vi "Day 22-Part 2-Split Cubes.vi"() -> ()   [LabVIEW 2021]
uses:
  <vilib>/regexp/Match Regular Expression.xnode
  <vilib>/Utility/file.llb/Read Delimited Spreadsheet (string).vi
panel:
  out "size(s)":i32[](array[numeric])
  out "Cubes On":i64
  out "Array":cluster{bool, i32[]}[](array[cluster])
  in  "Input File":enum32{"example input", "input"}(radio)
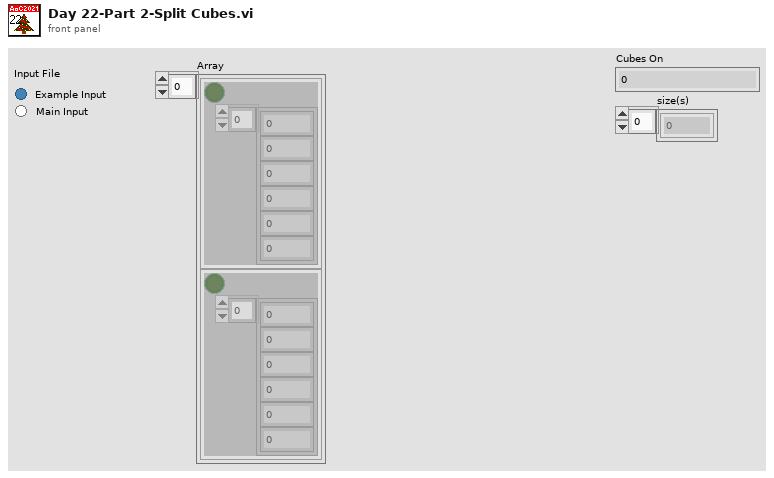
[diagram p1: front panel]
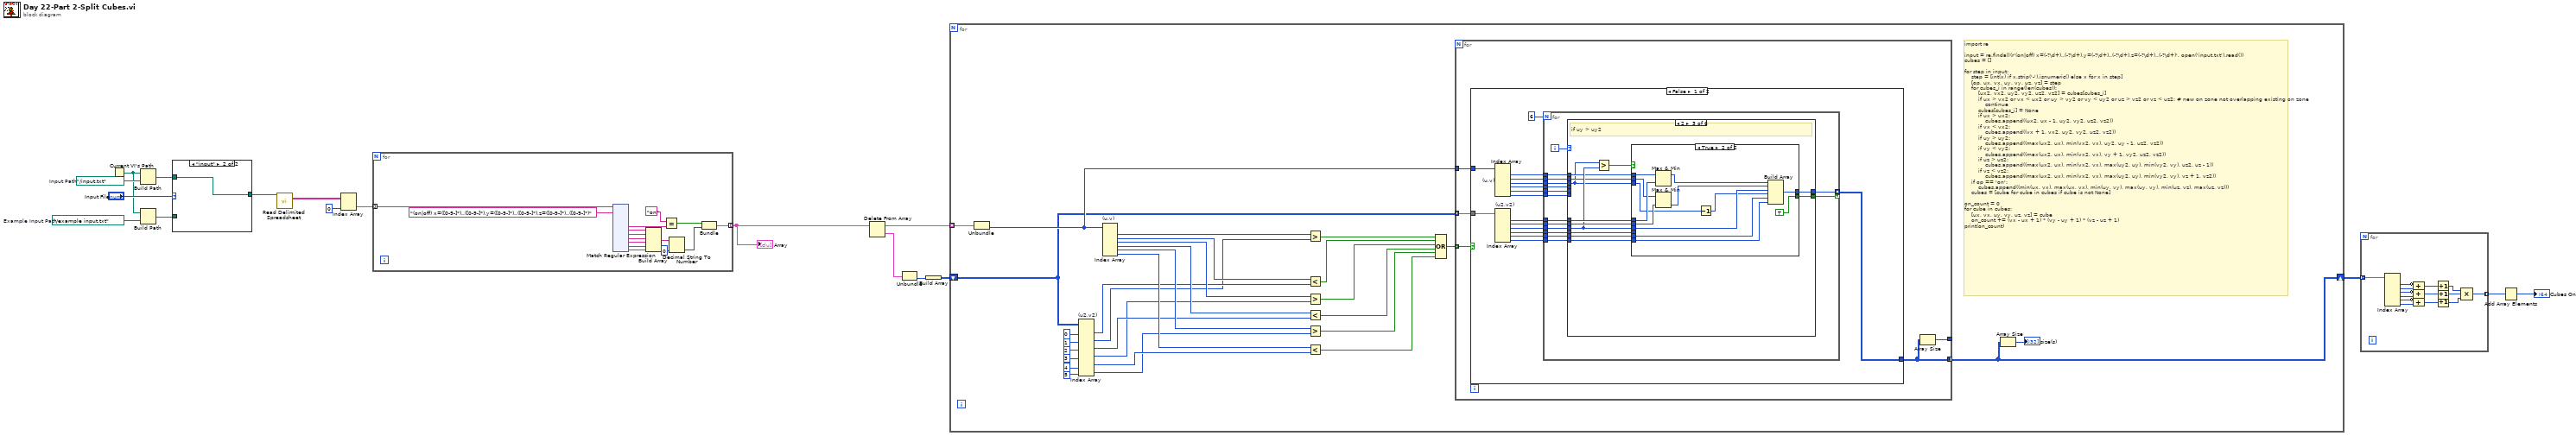
[diagram p0: block diagram]
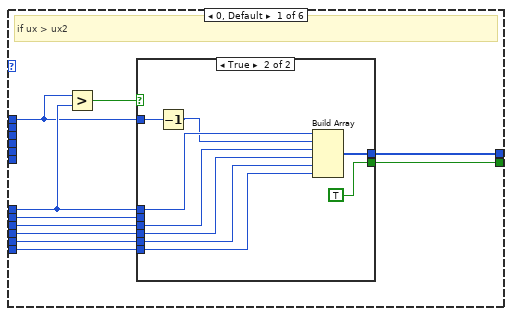
[diagram p2: hidden frame]
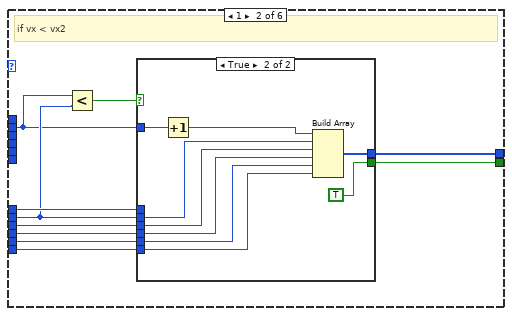
[diagram p4: hidden frame]
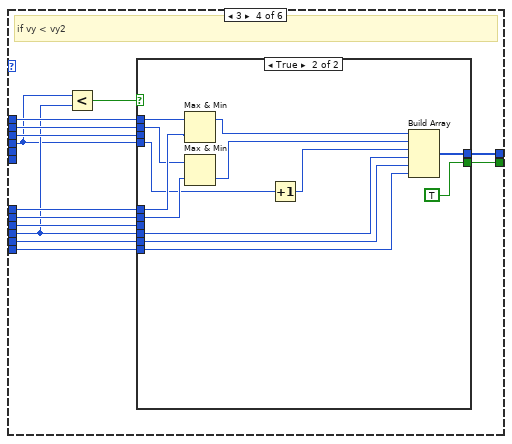
[diagram p7: hidden frame]
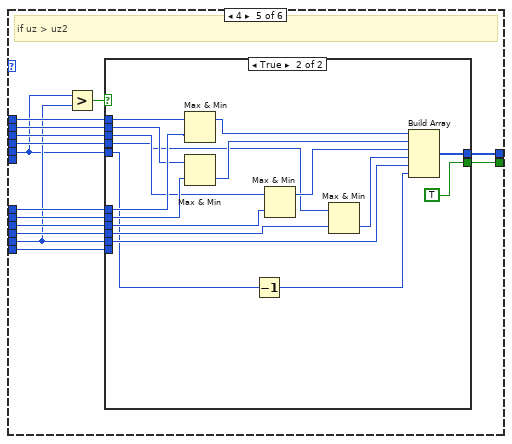
[diagram p9: hidden frame]
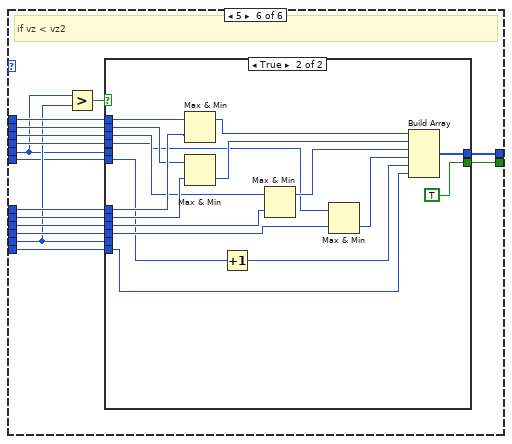
[diagram p11: hidden frame]
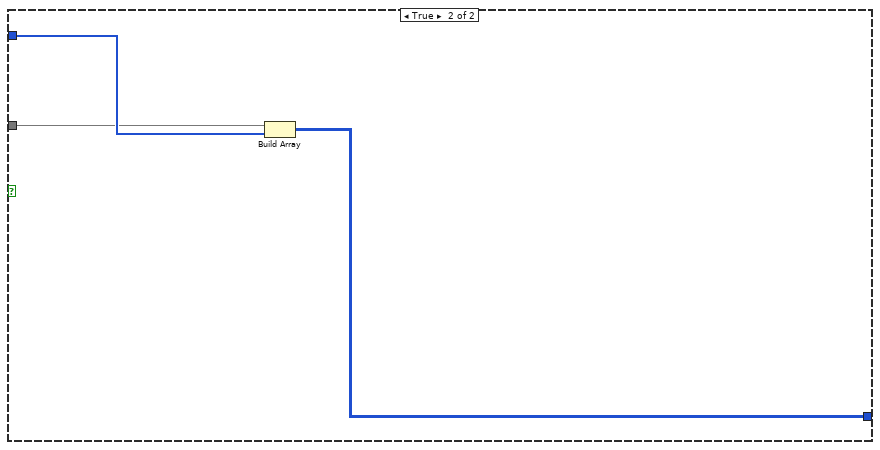
[diagram p13: hidden frame]
diagram:
  w17 = path "../example input.txt"  # Example Input Path
  w18 = path "../input.txt"  # Input Path
  n1 = Current VI's Path() -> (path=w12:path)
  n2 = Build Path(base path=w12, name or relative path=w18) -> (appended path=w15:path)
  n3 = Build Path(base path=w12, name or relative path=w17) -> (appended path=w14:path)
  n4 = case shown="\"input\"" "Input File" {
    tunnel: w15 -> [_ w20]
    tunnel: w14 -> [w19 _]
    tunnel: [w19 w20] -> w13
    frame "example input" {
    }
    frame "input" {
    }
  }
  n5 = call-poly <vilib>:"Read Delimited Spreadsheet.vi"("file path (dialog if empty)"=w13) -> ("all rows"=w11:string[][])  [unwired: 9 in, 5 out]
  n6 = Index Array(array=w11, index (col)=0 ("disabled index (col)")) -> (element=w9:string[])  [unwired: 1 in]
  n7 = for {
    tunnel: w9 -> [w35] mode=indexing
    tunnel: [w23] -> w8 mode=indexing
    n8 = xnode "Match Regular Expression"("input string"=w35, "regular expression"="(on|off) x=([0-9-]*)..([0-9-]*),y=([0-9-]*)..([0-9-]*),z=([0-9-]*)..([0-9-]*)") -> ("submatch 1"=w33:string, "submatch 2"=w30:string, "submatch 3"=w29:string, "submatch 4"=w28:string, "submatch 5"=w27:string, "submatch 6"=w26:string, "submatch 7"=w25:string)  [unwired: 4 in, 5 out]
    n9 = Build Array(w30, w29, w28, w27, w26, w25) -> (w24:string[])
    n10 = Equal?(x="on", y=w33) -> (x = y?=w31:bool)
    n11 = Decimal String To Number(string=w24, default (0L)=i64 0 ("default (0 I32)")) -> (number=w22:i64[])  [unwired: 1 in, 1 out]
    n12 = Bundle(w31, w22) -> (w23:cluster{bool, i64[]})  [unwired: 1 in]
  }
  "Array" <- w8
  n13 = Delete From Array(array=w8) -> (deleted portion=w6:cluster{bool, i64[]}, array with subset deleted=w7:cluster{bool, i64[]}[])  [unwired: 2 in]
  n14 = Unbundle(w6) -> (w5:i64[])  [unwired: 1 out]
  n15 = Build Array(w5) -> (w4:i64[][])
  n16 = for {
    tunnel: w7 -> [w190] mode=indexing
    shift-right: [w162] -> w3
    shift-left: w4 -> [w188]
    # "import re\n\ninput = re.findall(r'(on|off) x=(-?\\d+)..(-?\\d+),y=(-?\\d+)..(-?\\d+),z=(-?\\d+)..(-?\\d+)', open('input.txt').read())\ncubes = []\n\nfor step in input:\n    step = [int(x) if x.strip('-').isnumeric() else x for x in step]\n    [op, ux, vx, uy, vy, uz, vz] = step\n    for cubes_i in range(len(cubes)):\n        [ux2, vx2, uy2, vy2, uz2, vz2] = cubes[cubes_i]\n        if ux > vx2 or vx < ux2 or uy > vy2 or vy < uy2 or uz > vz2 or vz < uz2: # new on zone not overlapping existing on zone\n            continue\n        cubes[cubes_i] = None\n        if ux > ux2:\n            cubes.append((ux2, ux - 1, uy2, vy2, uz2, vz2))\n        if vx < vx2:\n            cubes.append((vx + 1, vx2, uy2, vy2, uz2, vz2))\n        if uy > uy2:\n            cubes.append((max(ux2, ux), min(vx2, vx), uy2, uy - 1, uz2, vz2))\n        if vy < vy2:\n            cubes.append((max(ux2, ux), min(vx2, vx), vy + 1, vy2, uz2, vz2))\n        if uz > uz2:\n            cubes.append((max(ux2, ux), min(vx2, vx), max(uy2, uy), min(vy2, vy), uz2, uz - 1))\n        if vz < vz2:\n            cubes.append((max(ux2, ux), min(vx2, vx), max(uy2, uy), min(vy2, vy), vz + 1, vz2))\n    if op == 'on':\n        cubes.append((min(ux, vx), max(ux, vx), min(uy, vy), max(uy, vy), min(uz, vz), max(uz, vz)))\n    cubes = [cube for cube in cubes if cube is not None]\n\non_count = 0\nfor cube in cubes:\n    [ux, vx, uy, vy, uz, vz] = cube\n    on_count += (vx - ux + 1) * (vy - uy + 1) * (vz - uz + 1)\nprint(on_count)"
    n17 = Unbundle(w190) -> (w189:i64[])  [unwired: 1 out]
    n18 = Index Array "(u2,v2)"(array=w188, index (col) #1=0 ("disabled index (col)"), index (col) #2=1 ("index (col)"), index (col) #3=2 ("index (col)"), index (col) #4=3 ("index (col)"), index (col) #5=4 ("index (col)"), index (col) #6=5 ("index (col)")) -> (element #1=w169:i64[], element #2=w168:i64[], element #3=w167:i64[], element #4=w166:i64[], element #5=w165:i64[], element #6=w164:i64[])  [unwired: 6 in]
    n19 = Index Array "(u,v)"(array=w189) -> (element #1=w187:i64, element #2=w185:i64, element #3=w183:i64, element #4=w181:i64, element #5=w179:i64, element #6=w178:i64)  [unwired: 6 in]
    n20 = Greater?(x=w187, y=w168) -> (0:w186:bool[])
    n21 = Less?(x=w185, y=w169) -> (x < y?=w184:bool[])
    n22 = Greater?(x=w183, y=w166) -> (0:w182:bool[])
    n23 = Less?(x=w181, y=w167) -> (x < y?=w180:bool[])
    n24 = Greater?(x=w179, y=w164) -> (0:w177:bool[])
    n25 = Less?(x=w178, y=w165) -> (x < y?=w176:bool[])
    n26 = Compound Arithmetic op=OR(w186, w184, w182, w180, w177, w176) -> (w163:bool[])
    n27 = for {
      tunnel: w189 -> [w195]
      tunnel: w188 -> [w194] mode=indexing
      tunnel: [w192] -> w162 mode=concatenating
      tunnel: w163 -> [w193] mode=indexing
      tunnel: [w191] -> _
      n28 = case shown="False" w193 {
        tunnel: w195 -> [w211 w381]
        tunnel: [w196 w380] -> w192
        tunnel: w194 -> [w210 w379]
        frame False {
          n29 = Index Array "(u,v)"(array=w211) -> (element #1=w209:i64, element #2=w201:i64, element #3=w200:i64, element #4=w199:i64, element #5=w198:i64, element #6=w197:i64)  [unwired: 6 in]
          n30 = Index Array "(u2,v2)"(array=w210) -> (element #1=w207:i64, element #2=w208:i64, element #3=w206:i64, element #4=w205:i64, element #5=w204:i64, element #6=w203:i64)  [unwired: 6 in]
          n31 = for {
            N: 6 -> [_]
            tunnel: w209 -> [w226]
            tunnel: w208 -> [w225]
            tunnel: w207 -> [w224]
            tunnel: w206 -> [w223]
            tunnel: w205 -> [w222]
            tunnel: w204 -> [w221]
            tunnel: w203 -> [w220]
            tunnel: w201 -> [w216]
            tunnel: w200 -> [w215]
            tunnel: w199 -> [w214]
            tunnel: w198 -> [w213]
            tunnel: w197 -> [w212]
            tunnel: [w218] -> w196 mode=indexing if=w217
            i -> [w219]
            n32 = case shown="2" w219 {
              tunnel: w226 -> [w229 _ w267 w294 w322 w354]
              tunnel: w225 -> [w235 w247 w269 w296 w324 w356]
              tunnel: w224 -> [w234 w254 w275 w301 w328 w360]
              tunnel: w223 -> [w233 w253 w268 w295 w323 w355]
              tunnel: w222 -> [w232 w252 w274 w291 w319 w351]
              tunnel: w221 -> [w231 w251 w273 w300 w317 w349]
              tunnel: w220 -> [w230 w250 w272 w299 w327 w359]
              tunnel: [w228 w249 w271 w298 w326 w358] -> w218
              tunnel: [w227 w248 w270 w297 w325 w357] -> w217
              tunnel: w216 -> [_ w246 w266 w293 w321 w353]
              tunnel: w215 -> [_ _ w265 w292 w320 w352]
              tunnel: w214 -> [_ _ _ w290 w318 w350]
              tunnel: w213 -> [_ _ _ _ w316 w348]
              tunnel: w212 -> [_ _ _ _ _ w347]
              frame 0, Default {
                # "if ux > ux2"
                n33 = Greater?(x=w229, y=w234) -> (0:w236:bool)
                n34 = case shown="True" w236 {
                  tunnel: w235 -> [_ _]
                  tunnel: w234 -> [_ w245]
                  tunnel: w233 -> [_ w242]
                  tunnel: w232 -> [_ w241]
                  tunnel: w231 -> [_ w240]
                  tunnel: w230 -> [_ w239]
                  tunnel: w229 -> [_ w244]
                  tunnel: [_ w238] -> w228
                  tunnel: [_ TRUE] -> w227
                  frame False {
                  }
                  frame True {
                    n35 = Decrement(x=w244) -> (x-1=w243:i64)
                    n36 = Build Array(w245, w243, w242, w241, w240, w239) -> (w238:i64[])
                  }
                }
              }
              frame 1 {
                # "if vx < vx2"
                n37 = Less?(x=w246, y=w247) -> (x < y?=w255:bool)
                n38 = case shown="True" w255 {
                  tunnel: w247 -> [_ w256]
                  tunnel: w254 -> [_ _]
                  tunnel: w253 -> [_ w264]
                  tunnel: w252 -> [_ w263]
                  tunnel: w251 -> [_ w262]
                  tunnel: w250 -> [_ w261]
                  tunnel: [_ w260] -> w249
                  tunnel: [_ TRUE] -> w248
                  tunnel: w246 -> [_ w258]
                  frame False {
                  }
                  frame True {
                    n39 = Increment(x=w258) -> (x+1=w257:i64)
                    n40 = Build Array(w257, w256, w264, w263, w262, w261) -> (w260:i64[])
                  }
                }
              }
              frame 2 {
                # "if uy > uy2"
                n41 = Greater?(x=w265, y=w268) -> (0:w276:bool)
                n42 = case shown="True" w276 {
                  tunnel: w269 -> [_ w279]
                  tunnel: w275 -> [_ w283]
                  tunnel: w268 -> [_ w289]
                  tunnel: w274 -> [_ _]
                  tunnel: w273 -> [_ w288]
                  tunnel: w272 -> [_ w287]
                  tunnel: [_ w286] -> w271
                  tunnel: [_ TRUE] -> w270
                  tunnel: w267 -> [_ w284]
                  tunnel: w266 -> [_ w281]
                  tunnel: w265 -> [_ w278]
                  frame False {
                  }
                  frame True {
                    n43 = Max & Min(x=w284, y=w283) -> (max(x,y)=w282:i64)  [unwired: 1 out]
                    n44 = Max & Min(x=w281, y=w279) -> (min(x,y)=w280:i64)  [unwired: 1 out]
                    n45 = Decrement(x=w278) -> (x-1=w277:i64)
                    n46 = Build Array(w282, w280, w289, w277, w288, w287) -> (w286:i64[])
                  }
                }
              }
              frame 3 {
                # "if vy < vy2"
                n47 = Less?(x=w290, y=w291) -> (x < y?=w302:bool)
                n48 = case shown="True" w302 {
                  tunnel: w296 -> [_ w306]
                  tunnel: w301 -> [_ w310]
                  tunnel: w295 -> [_ _]
                  tunnel: w291 -> [_ w303]
                  tunnel: w300 -> [_ w315]
                  tunnel: w299 -> [_ w314]
                  tunnel: [_ w313] -> w298
                  tunnel: [_ TRUE] -> w297
                  tunnel: w294 -> [_ w311]
                  tunnel: w293 -> [_ w308]
                  tunnel: w292 -> [_ _]
                  tunnel: w290 -> [_ w305]
                  frame False {
                  }
                  frame True {
                    n49 = Max & Min(x=w311, y=w310) -> (max(x,y)=w309:i64)  [unwired: 1 out]
                    n50 = Max & Min(x=w308, y=w306) -> (min(x,y)=w307:i64)  [unwired: 1 out]
                    n51 = Increment(x=w305) -> (x+1=w304:i64)
                    n52 = Build Array(w309, w307, w304, w303, w315, w314) -> (w313:i64[])
                  }
                }
              }
              frame 4 {
                # "if uz > uz2"
                n53 = Greater?(x=w316, y=w317) -> (0:w329:bool)
                n54 = case shown="True" w329 {
                  tunnel: w324 -> [_ w338]
                  tunnel: w328 -> [_ w342]
                  tunnel: w323 -> [_ w336]
                  tunnel: w319 -> [_ w333]
                  tunnel: w317 -> [_ w346]
                  tunnel: w327 -> [_ _]
                  tunnel: [_ w345] -> w326
                  tunnel: [_ TRUE] -> w325
                  tunnel: w322 -> [_ w343]
                  tunnel: w321 -> [_ w340]
                  tunnel: w320 -> [_ w337]
                  tunnel: w318 -> [_ w334]
                  tunnel: w316 -> [_ w331]
                  frame False {
                  }
                  frame True {
                    n55 = Max & Min(x=w343, y=w342) -> (max(x,y)=w341:i64)  [unwired: 1 out]
                    n56 = Max & Min(x=w340, y=w338) -> (min(x,y)=w339:i64)  [unwired: 1 out]
                    n57 = Decrement(x=w331) -> (x-1=w330:i64)
                    n58 = Max & Min(x=w337, y=w336) -> (max(x,y)=w335:i64)  [unwired: 1 out]
                    n59 = Max & Min(x=w334, y=w333) -> (min(x,y)=w332:i64)  [unwired: 1 out]
                    n60 = Build Array(w341, w339, w335, w332, w346, w330) -> (w345:i64[])
                  }
                }
              }
              frame 5 {
                # "if vz < vz2"
                n61 = Greater?(x=w348, y=w349) -> (0:w361:bool)
                n62 = case shown="True" w361 {
                  tunnel: w356 -> [_ w371]
                  tunnel: w360 -> [_ w375]
                  tunnel: w355 -> [_ w369]
                  tunnel: w351 -> [_ w366]
                  tunnel: w349 -> [_ _]
                  tunnel: w359 -> [_ w362]
                  tunnel: [_ w378] -> w358
                  tunnel: [_ TRUE] -> w357
                  tunnel: w354 -> [_ w376]
                  tunnel: w353 -> [_ w373]
                  tunnel: w352 -> [_ w370]
                  tunnel: w350 -> [_ w367]
                  tunnel: w348 -> [_ _]
                  tunnel: w347 -> [_ w364]
                  frame False {
                  }
                  frame True {
                    n63 = Max & Min(x=w376, y=w375) -> (max(x,y)=w374:i64)  [unwired: 1 out]
                    n64 = Max & Min(x=w373, y=w371) -> (min(x,y)=w372:i64)  [unwired: 1 out]
                    n65 = Increment(x=w364) -> (x+1=w363:i64)
                    n66 = Max & Min(x=w370, y=w369) -> (max(x,y)=w368:i64)  [unwired: 1 out]
                    n67 = Max & Min(x=w367, y=w366) -> (min(x,y)=w365:i64)  [unwired: 1 out]
                    n68 = Build Array(w374, w372, w368, w365, w363, w362) -> (w378:i64[])
                  }
                }
              }
            }
          }
        }
        frame True {
          n69 = Build Array(w379, w381) -> (w380:i64[][])
        }
      }
      n70 = Array Size(array=w192) -> (size(s)=w191:i32[])
    }
    n71 = Array Size(array=w162) -> (size(s)=→"size(s)":i32[])
  }
  n72 = for {
    tunnel: w3 -> [w395] mode=indexing
    tunnel: [w382] -> w1 mode=indexing
    n73 = Index Array(array=w395) -> (element #1=w394:i64, element #2=w393:i64, element #3=w392:i64, element #4=w391:i64, element #5=w390:i64, element #6=w389:i64)  [unwired: 6 in]
    n74 = Compound Arithmetic op=ADD(invert w394, w393) -> (w388:i64)
    n75 = Compound Arithmetic op=ADD(invert w392, w391) -> (w387:i64)
    n76 = Compound Arithmetic op=ADD(invert w390, w389) -> (w386:i64)
    n77 = Increment(x=w388) -> (x+1=w384:i64)
    n78 = Increment(x=w387) -> (x+1=w385:i64)
    n79 = Increment(x=w386) -> (x+1=w383:i64)
    n80 = Compound Arithmetic op=MULTIPLY(w384, w385, w383) -> (w382:i64)
  }
  n81 = Add Array Elements(numeric array=w1) -> (sum=→"Cubes On":i64)
